vi "Initialise DSP Queue.vi"(8 "error in (no error)":errorcluster) -> (0 "error out":errorcluster)   [LabVIEW 2016]
uses:
  Utilities/Application Globals.vi
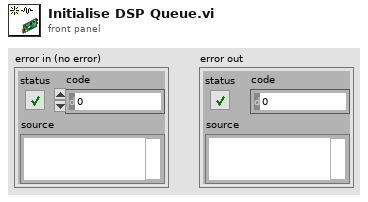
[diagram p1: front panel]
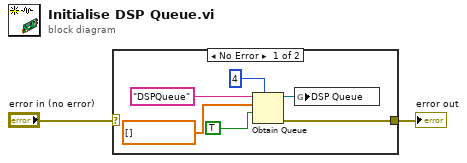
[diagram p0: block diagram]
diagram:
  n1 = case shown="No Error" "error in (no error)" {
    selector: "error in (no error)" -> [_ w9]
    tunnel: [w5 w9] -> w1
    frame No Error {
      n2 = Obtain Queue(max queue size (-1, unlimited)=4, name (unnamed)="DSPQueue", element data type=cdb[] [] ("x + iy"), create if not found? (T)=TRUE) -> (queue out=w3:refnum<queue>, error out=w5:errorcluster)  [unwired: 1 in, 1 out]
      n3 = global write "Application Globals.vi" "DSP Queue"(w3) -> ()
    }
    frame Error {
    }
  }
  "error out" <- w1
